vi "Control Panel.vi"(8 "error in (no error)":errorcluster, 11 "Keithley Multimeter in":refnum<class "Keithley Multimeter.lvclass">) -> (0 "error out":errorcluster, 3 "Keithley Multimeter out":refnum<class "Keithley Multimeter.lvclass">)   [LabVIEW 2023, in "Keithley Multimeter.lvclass"]
doc: "(Dynamic) A user-level application that simulates the physical front panel of the Instrument. Provide the user with buttons to manually control features of the instrument, and provide indicators of its current state."
uses:
  Keithley Multimeter.lvclass
  Keithley Multimeter.lvclass/Keithley Multimeter.ctl
panel:
  in  "Cont. Read":bool
  out "Unit":string="V"
  out "Current function":u16(ring)=1 items=["ac voltage", "dc voltage", "2-wire resistance", "4-wire resistance", "ac current", "dc current", "frequency", "temperature"]
  out "Tab Control":enum32{"0", "1", "2", "3", "4", "5", "6", "7"}(tab)
  in  "AC Voltage Configuration":T1={"dBm ref impedance (75:1)"=1, "peak window (secs)"=0.1, "detector (rms:0)"=0, "dB reference (volts)"=1.0, "AC voltage (volts:0)"=0, "reference value (volts)"=0.0, "range value (volts)"=750.0} {"range value (volts)" min=0.2 max=750.0 format="%^.2e"; "reference value (volts)" min=-775.0 max=775.0 format="%^.2e"; "AC voltage (volts:0)" items=["volts", "DB", "DBM"]; "dB reference (volts)" min=0.001 max=750.0 format="%.3f"; "detector (rms:0)" items=["RMS", "average", "low frequency RMS", "AC peak voltage", "DC negative peak spike", "DC positive peak spike"]; "peak window (secs)" min=0.1 max=9.9 format="%.2f"; "dBm ref impedance (75:1)" items=["50 ohms", "75 ohms", "93 ohms", "132 ohms", "300 ohms", "600 ohms"]}
  in  "DC Voltage Configuration":T2={"reference value (volts)"=0.0, "range value (volts)"=1000.0} {"range value (volts)" min=0.2 max=1000.0 format="%^.2e"; "reference value (volts)" min=-1100.0 max=1100.0 format="%^.2e"}
  in  "2 Wire Resistance Configuration":T3={"offset compensation"=FALSE, "reference value (ohms)"=0.0, "range value (ohms)"=1000000000.0} {"range value (ohms)" min=20.0 max=1000000000.0 format="%^.2e"; "reference value (ohms)" min=-1000000000.0 max=1000000000.0 format="%^.2e"}
  in  "4 Wire Resistance Configuration":T3={"offset compensation"=FALSE, "reference value (ohms)"=0.0, "range value (ohms)"=200000.0} {"range value (ohms)" min=20.0 max=200000.0 format="%^.2e"; "reference value (ohms)" min=-200000.0 max=200000.0 format="%^.2e"}
  in  "AC Current Configuration":T4={"detector (rms:0)"=0, "reference value (amps)"=0.0, "range value (amps)"=2.0} {"range value (amps)" min=0.0002 max=2.0 format="%^.2e"; "reference value (amps)" min=-2.1 max=2.1 format="%^.2e"; "detector (rms:0)" items=["RMS", "average"]}
  in  "DC Current Configuration":T5={"reference value (amps)"=0.0, "method"=TRUE, "range value (amps)"=2.0} {"range value (amps)" min=0.0002 max=2.0 format="%^.2e"; "reference value (amps)" min=-2.1 max=2.1 format="%^.2e"}
  in  "Frequency Configuration":T6={"source"=FALSE, "resolution (5 digits:1)"=1, "threshold current range (1mA:0)"=0, "reference value (Hz)"=0.0, "threshold current level"=0.0, "threshold voltage range (10V:1)"=1, "threshold voltage level"=0.0} {"threshold voltage level" min=-600.0 max=600.0 step=1.0 format="%^.2e"; "threshold voltage range (10V:1)" items=["1 V", "10 V", "100 V", "1000 V", "TTL"]; "threshold current level" min=-0.6 max=0.6 format="%^.2e"; "reference value (Hz)" min=0.0 max=15000000.0 format="%^.2e"; "threshold current range (1mA:0)" items=["1 mA", "10 mA", "100 mA", "1 A"]; "resolution (5 digits:1)" items=["4 digits", "5 digits"]}
  out "String":string
  in  "Configuration Values":T7={"range (auto:0)"=0, "dig. filter count"=10.0, "digital filter (off:0)"=0, "advanced filter (off:0)"=0, "integration time (0:auto)"=0, "integ. value"=0.01667, "resolution (4.5 digits:3)"=3, "noise tolerance (%)"=1.0, "reference (off:0)"=0, "coupling"=TRUE, "function (Vdc:1)"=1} {"function (Vdc:1)" items=["ac voltage", "dc voltage", "2-wire resistance", "4-wire resistance", "ac current", "dc current", "frequency", "temperature"]; "reference (off:0)" items=["off", "set reference value"]; "noise tolerance (%)" min=0.0 max=100.0 step=1.0 format="%^.2e"; "resolution (4.5 digits:3)" items=["auto resolution", "auto resolution once", "3.5 digits", "4.5 digits", "5.5 digits", "6.5 digits", "7.5 digits", "8.5 digits"]; "integ. value" format="%^.2e"; "integration time (0:auto)" items=["automatic", "automatic once", "set to minimum", "set to maximum", "set aperature value", "set NPLC value"]; "advanced filter (off:0)" items=["off", "enabled"]; "digital filter (off:0)" items=["off", "auto filter", "auto filter once", "moving filter", "repeating filter"]; "dig. filter count" min=1.0 max=100.0 step=1.0 format="%^.2e"; "range (auto:0)" items=["autorange", "autorange once", "set min range", "set max range", "set range value"]}
  in  "function (Vdc:1)":u16(ring)=1 items=["ac voltage", "dc voltage", "2-wire resistance", "4-wire resistance", "ac current", "dc current", "frequency", "temperature"]
  in  "Set":bool
  in  "Read":bool
  out "Output":dbl[](array[numeric])
  in  "Stop":bool
  # "Doesn't work yet"
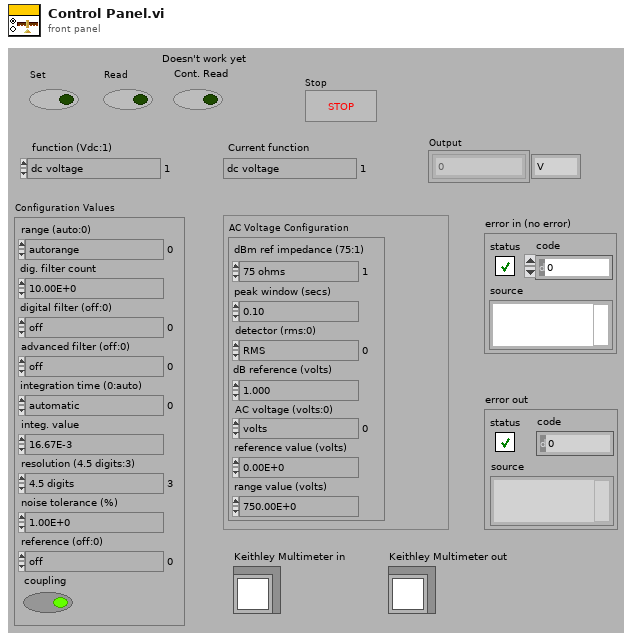
[diagram p1: front panel]
types:
  T1 = cluster{"dBm ref impedance (75:1)":u16, "peak window (secs)":dbl, "detector (rms:0)":u16, "dB reference (volts)":dbl, "AC voltage (volts:0)":u16, "reference value (volts)":dbl, "range value (volts)":dbl}
  T2 = cluster{"reference value (volts)":dbl, "range value (volts)":dbl}
  T3 = cluster{"offset compensation":bool, "reference value (ohms)":dbl, "range value (ohms)":dbl}
  T4 = cluster{"detector (rms:0)":u16, "reference value (amps)":dbl, "range value (amps)":dbl}
  T5 = cluster{"reference value (amps)":dbl, "method":bool, "range value (amps)":dbl}
  T6 = cluster{"source":bool, "resolution (5 digits:1)":u16, "threshold current range (1mA:0)":u16, "reference value (Hz)":dbl, "threshold current level":dbl, "threshold voltage range (10V:1)":u16, "threshold voltage level":dbl}
  T7 = cluster{"range (auto:0)":u16, "dig. filter count":dbl, "digital filter (off:0)":u16, "advanced filter (off:0)":u16, "integration time (0:auto)":u16, "integ. value":dbl, "resolution (4.5 digits:3)":u16, "noise tolerance (%)":dbl, "reference (off:0)":u16, "coupling":bool, "function (Vdc:1)":u16}
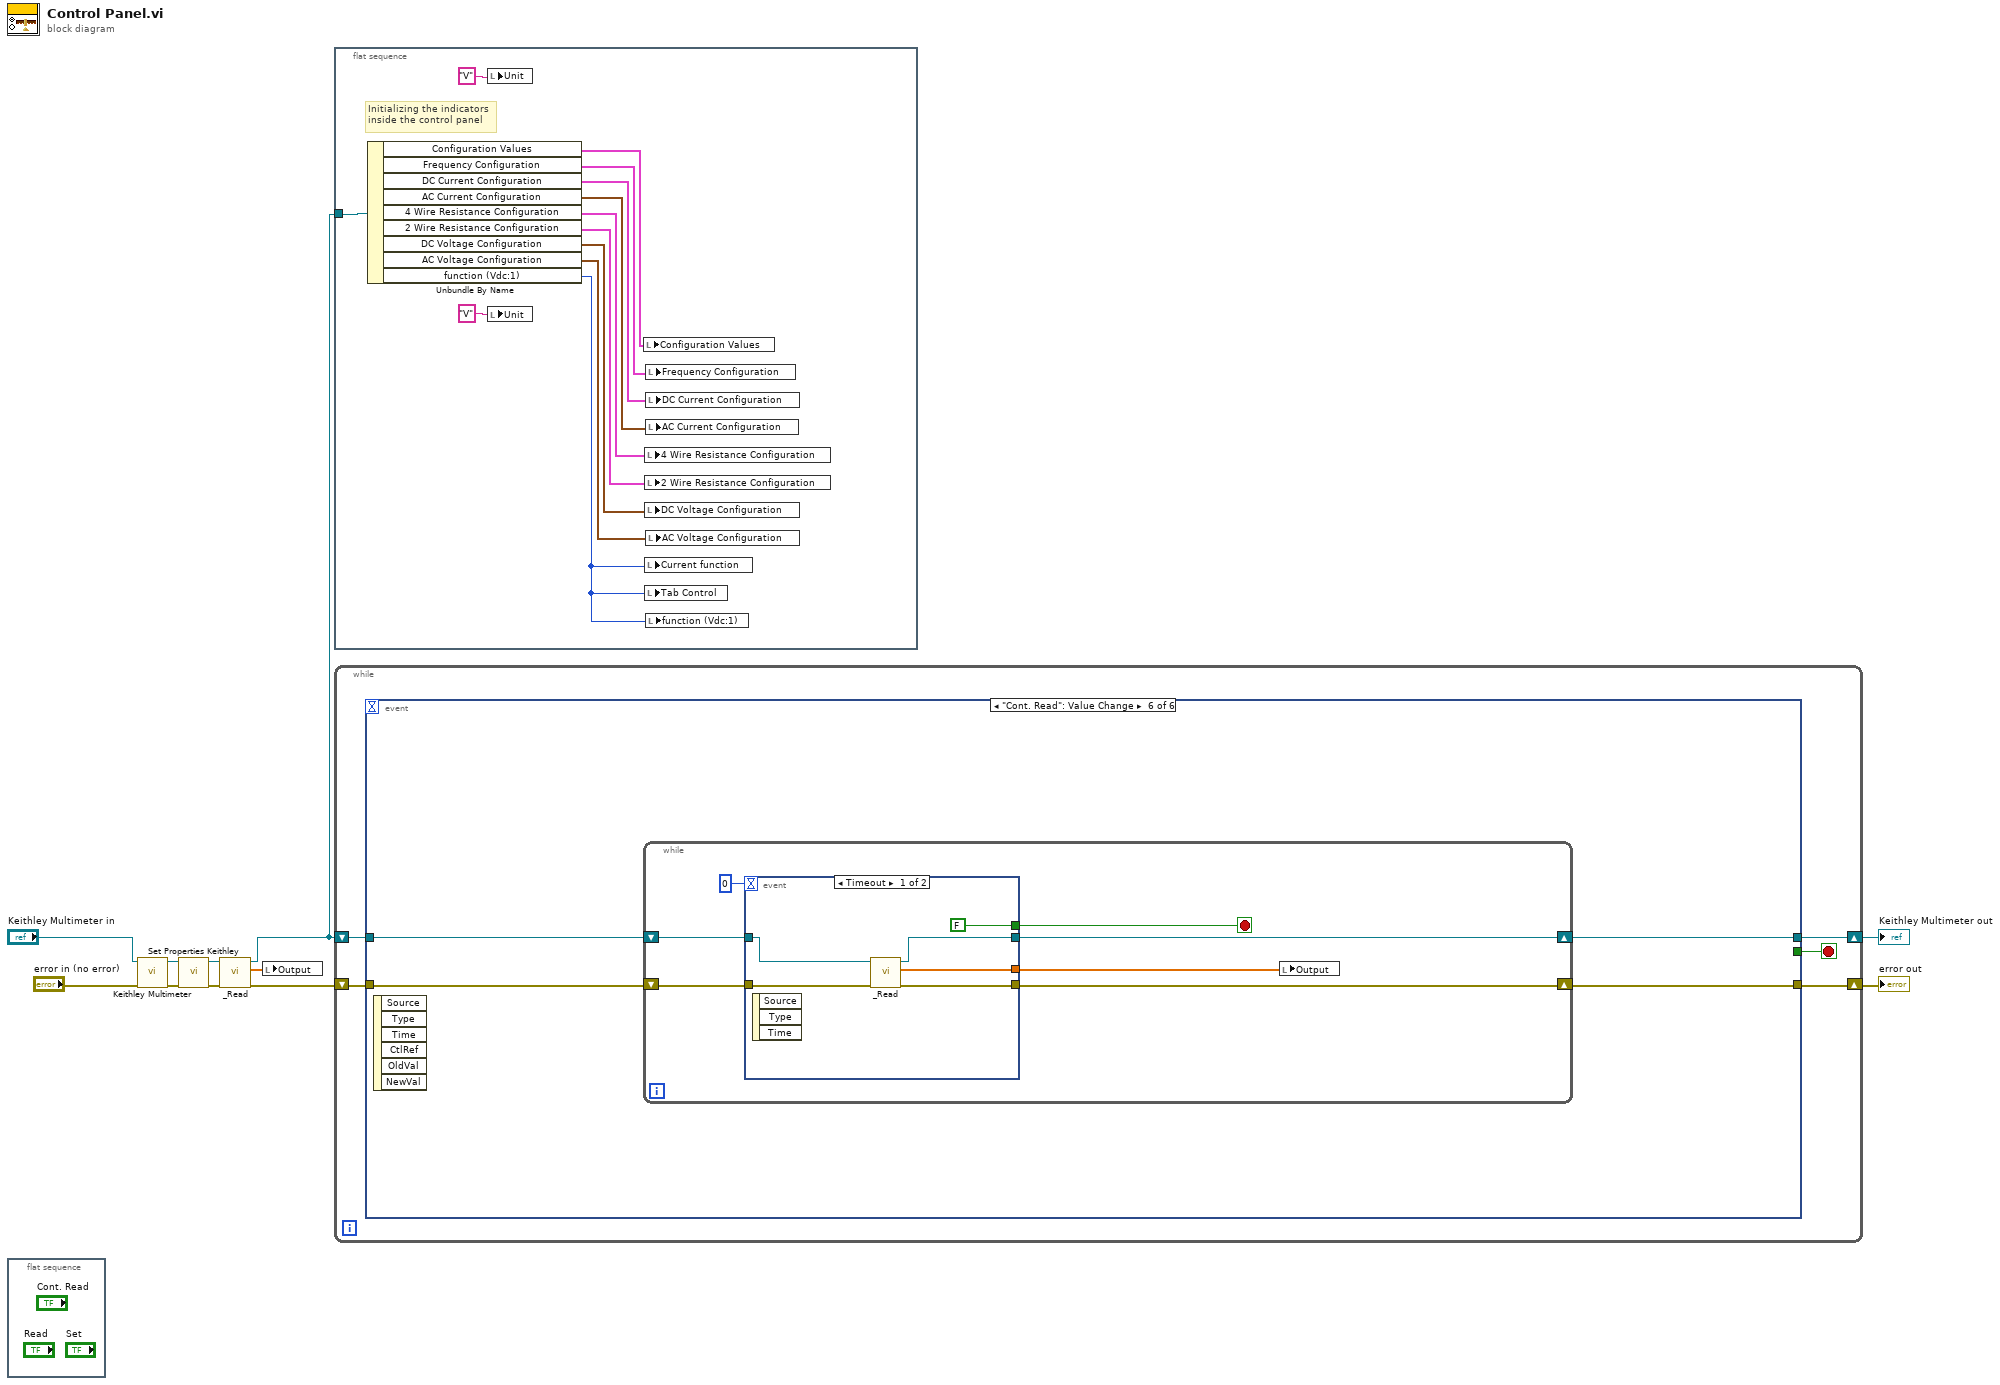
[diagram p0: block diagram]
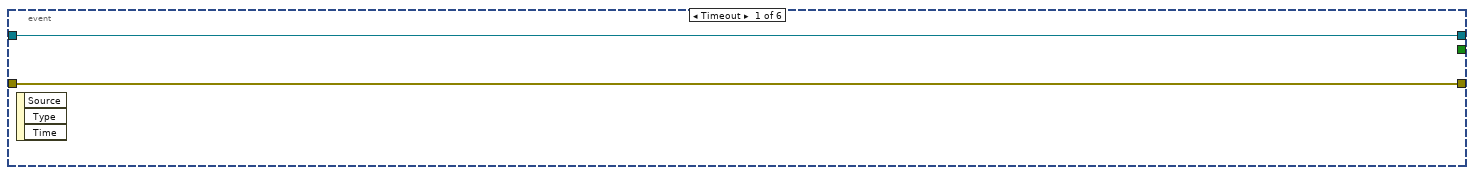
[diagram p2: hidden frame]
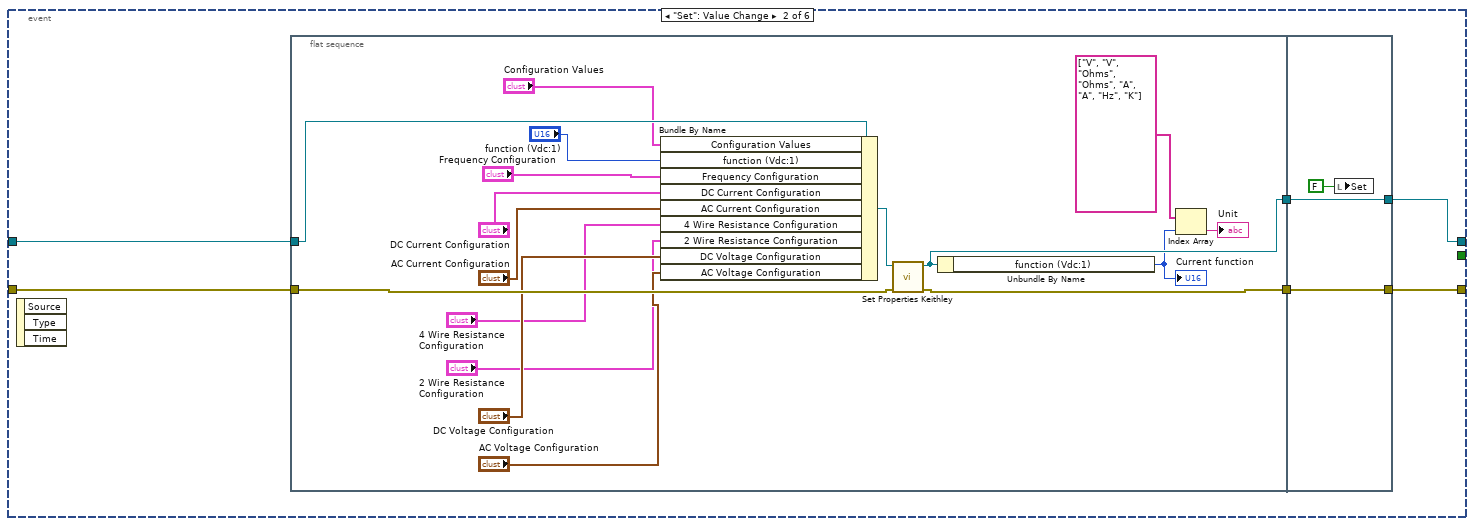
[diagram p3: hidden frame]
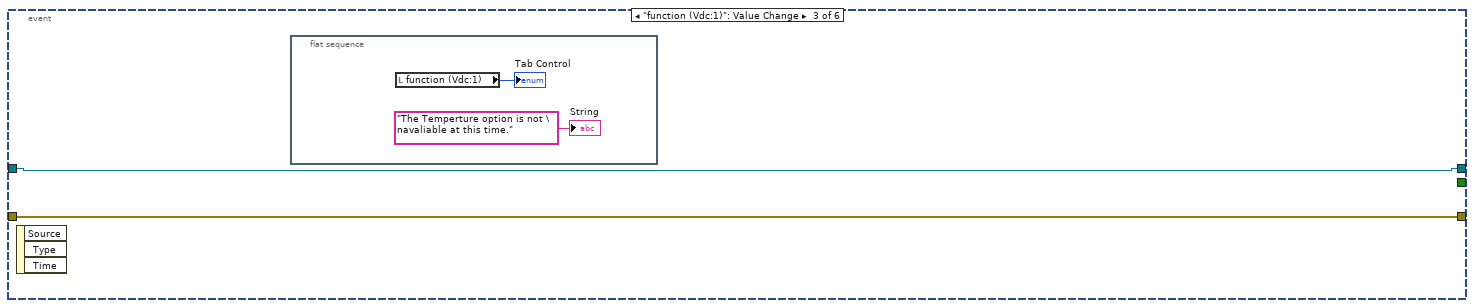
[diagram p4: hidden frame]
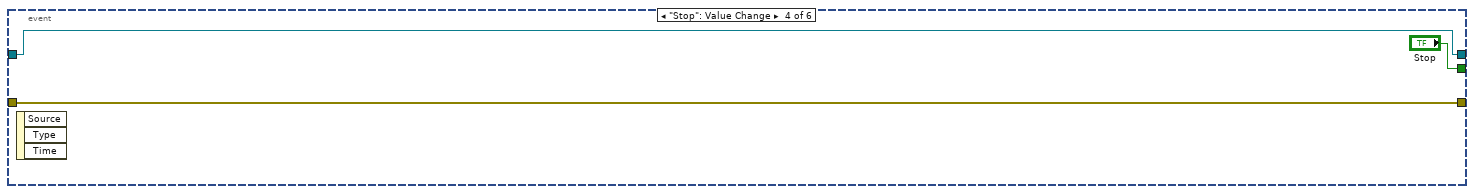
[diagram p5: hidden frame]
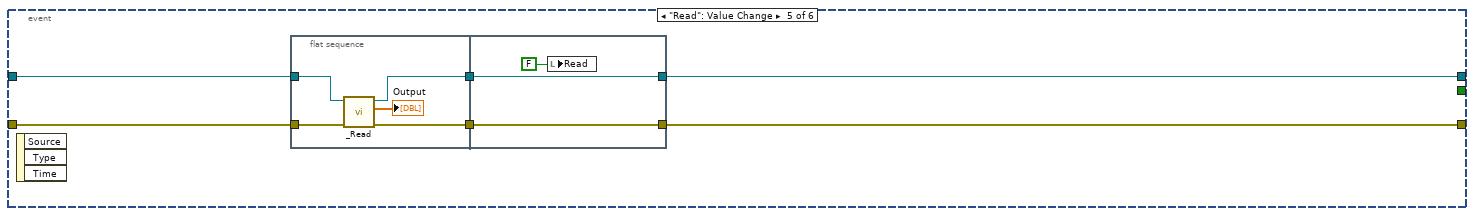
[diagram p6: hidden frame]
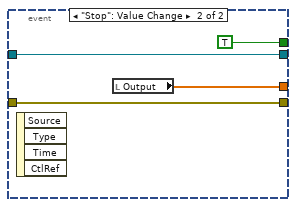
[diagram p7: hidden frame]
diagram:
  n1 = flat-sequence {
    frame #0 {
    }
  }
  n2 = call "Keithley Multimeter.vi"("error in (no error)"="error in (no error)", "Keithley Multimeter in"="Keithley Multimeter in") -> ("error out"=w8:errorcluster, "Keithley Multimeter out"=w7:refnum<class "Keithley Multimeter.lvclass">)  [unwired: 8 in]
  n3 = call-dynamic "Set Properties Keithley.vi"("error in (no error)"=w8, "Keithley Multimeter in"=w7) -> ("error out"=w4:errorcluster, "Keithley Multimeter out"=w5:refnum<class "Keithley Multimeter.lvclass">)  [unwired: 8 in]
  n4 = call-dynamic "_Read.vi"("error in (no error)"=w4, "Keithley Multimeter in"=w5) -> ("error out"=w3:errorcluster, "appended array"=w6:dbl[], "Keithley Multimeter out"=w2:refnum<class "Keithley Multimeter.lvclass">)  [unwired: 7 in]
  n5 = local write "Output"(w6) -> ()
  n6 = flat-sequence {
    tunnel: w2 -> [w23]
    frame #0 {
      # "Initializing the indicators\ninside the control panel"
      n7 = Unbundle By Name(w23) -> ("Configuration Values"=w22:T7, "Frequency Configuration"=w21:T6, "DC Current Configuration"=w19:T5, "AC Current Configuration"=w20:T4, "4 Wire Resistance Configuration"=w18:T3, "2 Wire Resistance Configuration"=w17:T3, "DC Voltage Configuration"=w16:T2, "AC Voltage Configuration"=w15:T1, "function (Vdc:1)"=w12:u16)
      n8 = local write "Unit"("V" ("Unit")) -> ()
      n9 = local write "Unit"("V" ("Unit")) -> ()
      n10 = local write "Configuration Values"(w22) -> ()
      n11 = local write "4 Wire Resistance Configuration"(w18) -> ()
      n12 = local write "2 Wire Resistance Configuration"(w17) -> ()
      n13 = local write "DC Voltage Configuration"(w16) -> ()
      n14 = local write "Current function"(w12) -> ()
      n15 = local write "Tab Control"(w12) -> ()
      n16 = local write "Frequency Configuration"(w21) -> ()
      n17 = local write "DC Current Configuration"(w19) -> ()
      n18 = local write "AC Current Configuration"(w20) -> ()
      n19 = local write "AC Voltage Configuration"(w15) -> ()
      n20 = local write "function (Vdc:1)"(w12) -> ()
    }
  }
  n21 = while {
    shift-right: [w27] -> w11
    shift-left: w2 -> [w25]
    shift-right: [w24] -> w1
    shift-left: w3 -> [w28]
    stop <- w26 stop-if-true
    n22 = event shown="[5] \"Cont. Read\": Value Change" {
      selector: _ -> [_ _ _ _ _ _]
      dyn-events: _ -> [_ _ _ _ _ _]
      timeout: _ -> [_ _ _ _ _ _]
      tunnel: w28 -> [w29 w33 w58 w61 w69 w80]
      tunnel: w25 -> [w30 w36 w57 w62 w68 w81]
      tunnel: [w29 w34 w58 w61 w67 w78] -> w24
      tunnel: [w30 w35 w57 w62 w66 w79] -> w27
      tunnel: [_ _ _ "Stop" _ _] -> w26
      event Timeout {
        n23 = event-data() -> ()  [unwired: 1 in, 3 out]
      }
      event "Set": Value Change {
        n24 = event-data() -> ()  [unwired: 1 in, 3 out]
        n25 = flat-sequence {
          tunnel: w36 -> [w53]
          tunnel: w33 -> [w49]
          tunnel: [w52] -> w32
          tunnel: [w50] -> w31
          tunnel: [w55] -> w34
          tunnel: [w56] -> w35
          tunnel: w32 -> [w56]
          tunnel: w31 -> [w55]
          frame #0 {
            n26 = Bundle By Name(cluster=w53, "Configuration Values"="Configuration Values", "function (Vdc:1)"="function (Vdc:1)", "Frequency Configuration"="Frequency Configuration", "DC Current Configuration"="DC Current Configuration", "AC Current Configuration"="AC Current Configuration", "4 Wire Resistance Configuration"="4 Wire Resistance Configuration", "2 Wire Resistance Configuration"="2 Wire Resistance Configuration", "DC Voltage Configuration"="DC Voltage Configuration", "AC Voltage Configuration"="AC Voltage Configuration") -> (w51:refnum<class "Keithley Multimeter.lvclass">)
            n27 = call-dynamic "Set Properties Keithley.vi"("error in (no error)"=w49, "Keithley Multimeter in"=w51) -> ("error out"=w50:errorcluster, "Keithley Multimeter out"=w52:refnum<class "Keithley Multimeter.lvclass">)  [unwired: 8 in]
            n28 = Unbundle By Name(w52) -> ("function (Vdc:1)"=w37:u16)
            "Current function" <- w37
            n29 = Index Array(array=string[] ["V", "V", "Ohms", "Ohms", "A", "A", "Hz", "K"], index=w37) -> (element=→"Unit":string)
          }
          frame #1 {
            n30 = local write "Set"(FALSE ("Set")) -> ()
          }
        }
      }
      event "function (Vdc:1)": Value Change {
        n31 = event-data() -> ()  [unwired: 1 in, 3 out]
        n32 = flat-sequence {
          frame #0 {
            n33 = local read "function (Vdc:1)"() -> (→"Tab Control":u16)
            "String" <- "The Temperture option is not \navaliable at this time." ("String")
          }
        }
      }
      event "Stop": Value Change {
        n34 = event-data() -> ()  [unwired: 1 in, 3 out]
      }
      event "Read": Value Change {
        n35 = event-data() -> ()  [unwired: 1 in, 3 out]
        n36 = flat-sequence {
          tunnel: w69 -> [w74]
          tunnel: w68 -> [w73]
          tunnel: [w72] -> w65
          tunnel: [w70] -> w64
          tunnel: [w76] -> w66
          tunnel: [w77] -> w67
          tunnel: w65 -> [w77]
          tunnel: w64 -> [w76]
          frame #0 {
            n37 = call-dynamic "_Read.vi"("error in (no error)"=w74, "Keithley Multimeter in"=w73) -> ("error out"=w72:errorcluster, "appended array"=→"Output":dbl[], "Keithley Multimeter out"=w70:refnum<class "Keithley Multimeter.lvclass">)  [unwired: 7 in]
          }
          frame #1 {
            n38 = local write "Read"(FALSE ("Read")) -> ()
          }
        }
      }
      event "Cont. Read": Value Change {
        n39 = event-data() -> ()  [unwired: 1 in, 6 out]
        n40 = while {
          shift-right: [w85] -> w78
          shift-left: w80 -> [w87]
          shift-right: [w86] -> w79
          shift-left: w81 -> [w88]
          stop <- w83 stop-if-true
          n41 = event shown="[0] Timeout" {
            selector: _ -> [_ _]
            dyn-events: _ -> [_ _]
            timeout: 0 -> [_ _]
            tunnel: w88 -> [w94 w98]
            tunnel: w87 -> [w93 w97]
            tunnel: [w92 w98] -> w86
            tunnel: [w91 w97] -> w85
            tunnel: [FALSE TRUE] -> w83
            tunnel: [w89 w95] -> w82
            event Timeout {
              n42 = event-data() -> ()  [unwired: 1 in, 3 out]
              n43 = call-dynamic "_Read.vi"("error in (no error)"=w93, "Keithley Multimeter in"=w94) -> ("error out"=w91:errorcluster, "appended array"=w89:dbl[], "Keithley Multimeter out"=w92:refnum<class "Keithley Multimeter.lvclass">)  [unwired: 7 in]
            }
            event "Stop": Value Change {
              n44 = event-data() -> ()  [unwired: 1 in, 4 out]
              n45 = local read "Output"() -> (w95:dbl[])
            }
          }
          n46 = local write "Output"(w82) -> ()
        }
      }
    }
  }
  "error out" <- w1
  "Keithley Multimeter out" <- w11
